vi "Device Select.vi"(8 "error in":errorcluster, 10 "SQL query":string="SELECT distinct DeviceName \nFROM\nltt.daq_configuration\n Where ChannelType='Digital_Output' and Enabled=1;", 11 "NI Digital Output in":refnum<class "NI Digital Output.lvclass">) -> (0 "error out":errorcluster, 3 "NI Digital Output out":refnum<class "NI Digital Output.lvclass">)   [LabVIEW 2023, in "HardwareAbstractionLayer_LVOOP.lvlib" / "NI Digital Output.lvclass"]
doc: "This VI Selected Device"
uses:
  NI Digital Output.lvclass
  NI Digital Output.lvclass/NI Digital Output.ctl
  Database/Database.lvclass
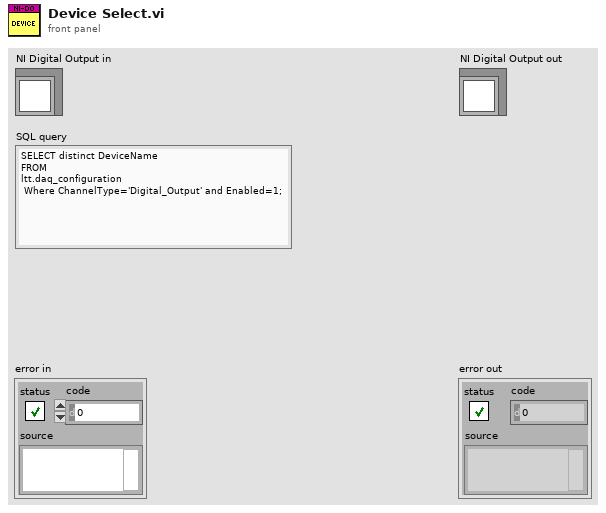
[diagram p1: front panel]
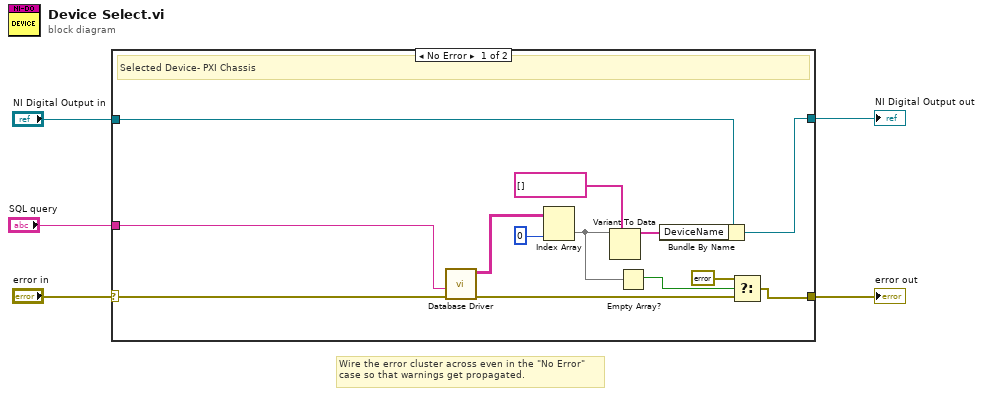
[diagram p0: block diagram]
diagram:
  # "Wire the error cluster across even in the \"No Error\"\ncase so that warnings get propagated."
  n1 = case shown="No Error" "error in" {
    selector: "error in" -> [w12 w20]
    tunnel: [w7 w20] -> w4
    tunnel: [w17 w19] -> w2
    tunnel: "NI Digital Output in" -> [w18 w19]
    tunnel: "SQL query" -> [w11 _]
    frame No Error {
      # "Selected Device- PXI Chassis"
      n2 = call "Database Driver.vi"("error in"=w12, "SQL query"=w11) -> ("error out"=w8:errorcluster, "data"=w13:string[][])  [unwired: 6 in, 2 out]
      n3 = Index Array(array=w13, index (col)=0 ("disabled index (col)")) -> (element=w10:string[])  [unwired: 1 in]
      n4 = Variant To Data(type=tag[] [] ("DeviceName"), Variant=w10) -> (data=w14:tag[])  [unwired: 1 in, 1 out]
      n5 = Empty Array?(array=w10) -> (empty?=w9:bool)
      n6 = Bundle By Name(cluster=w18, "DeviceName"=w14) -> (w17:refnum<class "NI Digital Output.lvclass">)
      n7 = Select(t=errorcluster {"status"=TRUE, "code"=0, "source"="Database does not contains device which is query."}, s=w9, f=w8) -> (s? t:f=w7:errorcluster)
    }
    frame Error {
    }
  }
  "error out" <- w4
  "NI Digital Output out" <- w2
